vi "testGetViRelease.vi"(8 "error in (no error)":errorcluster) -> (0 "error out":errorcluster)   [LabVIEW 2018]
uses:
  src/LibReader/LibReader.lvclass
  <vilib>/addons/_JKI Toolkits/Caraya/classes/Assert/Assert Equal Value_Variant.vi
  <vilib>/addons/_JKI Toolkits/Caraya/classes/Test/Test.lvclass
  <vilib>/addons/_JKI Toolkits/Caraya/classes/Assert/Assert.lvclass
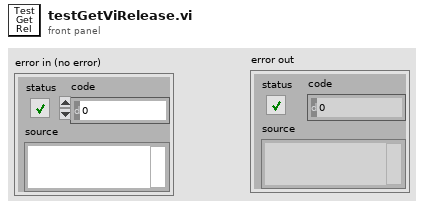
[diagram p1: front panel]
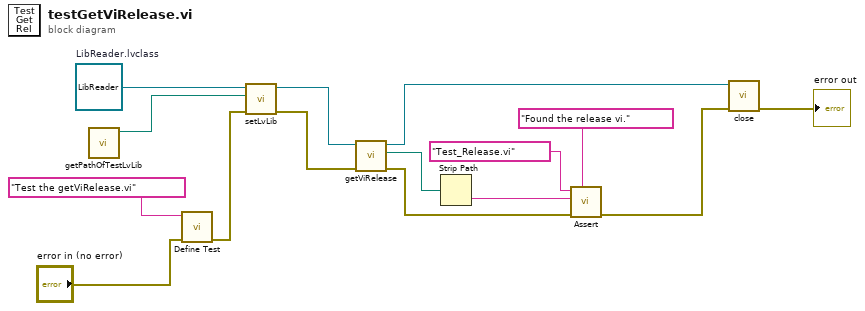
[diagram p0: block diagram]
diagram:
  w13 = refnum<class "LibReader.lvclass"> refnum  # LibReader.lvclass
  n1 = call "getPathOfTestLvLib.vi"() -> ("testLvLibPath"=w12:path)  [unwired: 11 in]
  n2 = call <vilib>:"Define Test.vi"("error in (no error)"="error in (no error)", "Label (VI Title)"="Test the getViRelease.vi") -> ("error out"=w11:errorcluster)  [unwired: 9 in]
  n3 = call "setLvLib.vi"("error in (no error)"=w11, "pathLvLib"=w12, "LibReader in"=w13) -> ("error out"=w9:errorcluster, "LibReader out"=w10:refnum<class "LibReader.lvclass">)  [unwired: 7 in]
  n4 = call "getViRelease.vi"("error in (no error)"=w9, "LibReader in"=w10) -> ("error out"=w5:errorcluster, "pathViRelease"=w7:path, "LibReader out"=w8:refnum<class "LibReader.lvclass">)  [unwired: 7 in]
  n5 = Strip Path(path=w7) -> (name=w6:string)  [unwired: 1 out]
  n6 = call-poly <vilib>:"Assert.vi"("Label"="Found the release vi.", "error in (no error)"=w5, "Y"=w6, "X"="Test_Release.vi") -> ("error out"=w4:errorcluster)  [unwired: 7 in]
  n7 = call "close.vi"("error in (no error)"=w4, "LibReader in"=w8) -> ("error out"=→"error out":errorcluster)  [unwired: 8 in, 1 out]
